vi "DataCollectTLSubs.vi"() -> ()   [LabVIEW 2009]
uses:
  BaudRateSelector.ctl
  <vilib>/Platform/TimedLoop/XDataNode/XDataNode.xnode
  <vilib>/Platform/TimedLoop/XDataNode/loadlvalarms.vi
  <vilib>/Platform/TimedLoop/XDataNode/timing_clust.ctl
  <vilib>/Platform/TimedLoop/XDataNode/nitl_modes.ctl
  <vilib>/Platform/TimedLoop/XDataNode/wakeup.ctl
  <vilib>/Platform/TimedLoop/scheduler/LVUserAPI/_suppVIs/Create_1kHz_TSource.vi
  <vilib>/Platform/TimedLoop/XDataNode/XDNodeRunTimeDep.lvlib
  <vilib>/Instr/_visa.llb/VISA Configure Serial Port (Instr).vi
panel:
  out "Sensor Names":string[](array[string])
  out "Degrees":dbl[](array[numeric]) format="%7.2f"
  in  "LH Calibration File":path
  out "Raw Data":u8[](array[numeric])
  out "Array 2":u32[](array[numeric])
  in  "Sampling Frequency (Hz)":u32 max=120 step=1
  in  "RH COM Port":refnum<visa-resource-name>="COM2"
  in  "LH COM Port":refnum<visa-resource-name>="COM1"
  out "Titles":string[](array[string])
  out "In queue":i32
  out "Interpreted Values":sgl[](array[numeric]) format="%.2f"
  out "Array":u32[](array[numeric])
  in  "stop":bool
  in  "Parity":enum16{"None", "Odd", "Even", "Mark", "Space"}(ring)
  in  "Data Bits":u16=8 min=7 max=8 step=1
  in  "Baud Rate":T1=115200 items=["1200"=1200, "2400"=2400, "4800"=4800, "9600"=9600, "19200"=19200, "38400"=38400, "57600"=57600, "115200"=115200]
  in  "COM Port":refnum<visa-resource-name>="COM3"
  # "Polhemus Serial Information"
  # "If Data Bits = 8, Parity must be \"None\""
  # "0 = As fast as possible"
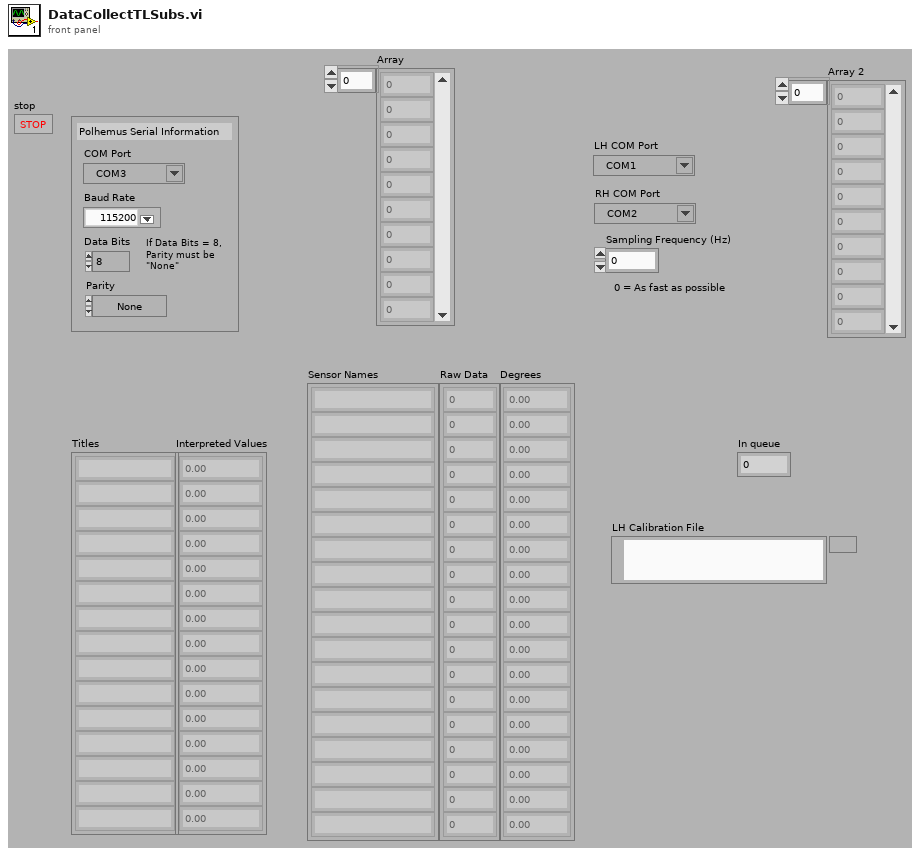
[diagram p1: front panel]
types:
  T1 = typedef "BaudRateSelector.ctl" = u32
  T2 = cluster{"#Bytes":i32[], "Titles":string[], "Format":enum16{"ASCII", "Binary"}, "Units":enum16{"Inches", "Centimeters"}, "Station State":bool[], "#Line Feeds":i32}
  T3 = typedef "XDNodeRunTimeDep.lvlib/timing_clust.ctl" = cluster{"Expected End [f-1]":u64, "Actual End [f-1]":u64, "Finished Late? [f-1]":bool, "Expected End [i-1]":u64, "Actual End [i-1]":u64, "Finished Late? [i-1]":bool, "Expected Start [i]":u64, "Actual Start [i]":u64, "Expected Start [f]":u64, "Actual Start [f]":u64, "Source Name":string, "Structure Name":string, "Period":i64, "Deadline":i64, "Offset":i64, "Start":i64, "Priority":i32, "Timeout":i32, "Mode":T4, "Wakeup Reason":T5, "Error":errorcluster, "Source Type":string, "Secondary Source Type":string, "Global End Time":u64, "Global Start Time":u64, "Frame Duration":u64, "Iteration Duration":u64, "Assigned CPU":i32, "I/O Scan Engine Mode":u32}
  T4 = typedef "XDNodeRunTimeDep.lvlib/nitl_modes.ctl" = enum32{"No Change", "Process missed periods, maintain original phase", "Discard missed periods, maintain original phase", "Process missed periods, ignore original phase", "Discard missed periods, ignore original phase"}
  T5 = typedef "XDNodeRunTimeDep.lvlib/wakeup.ctl" = enum32{"Normal", "Aborted", "Asynchronous wakeup", "Timing source error", "Timed loop error", "Timeout"}
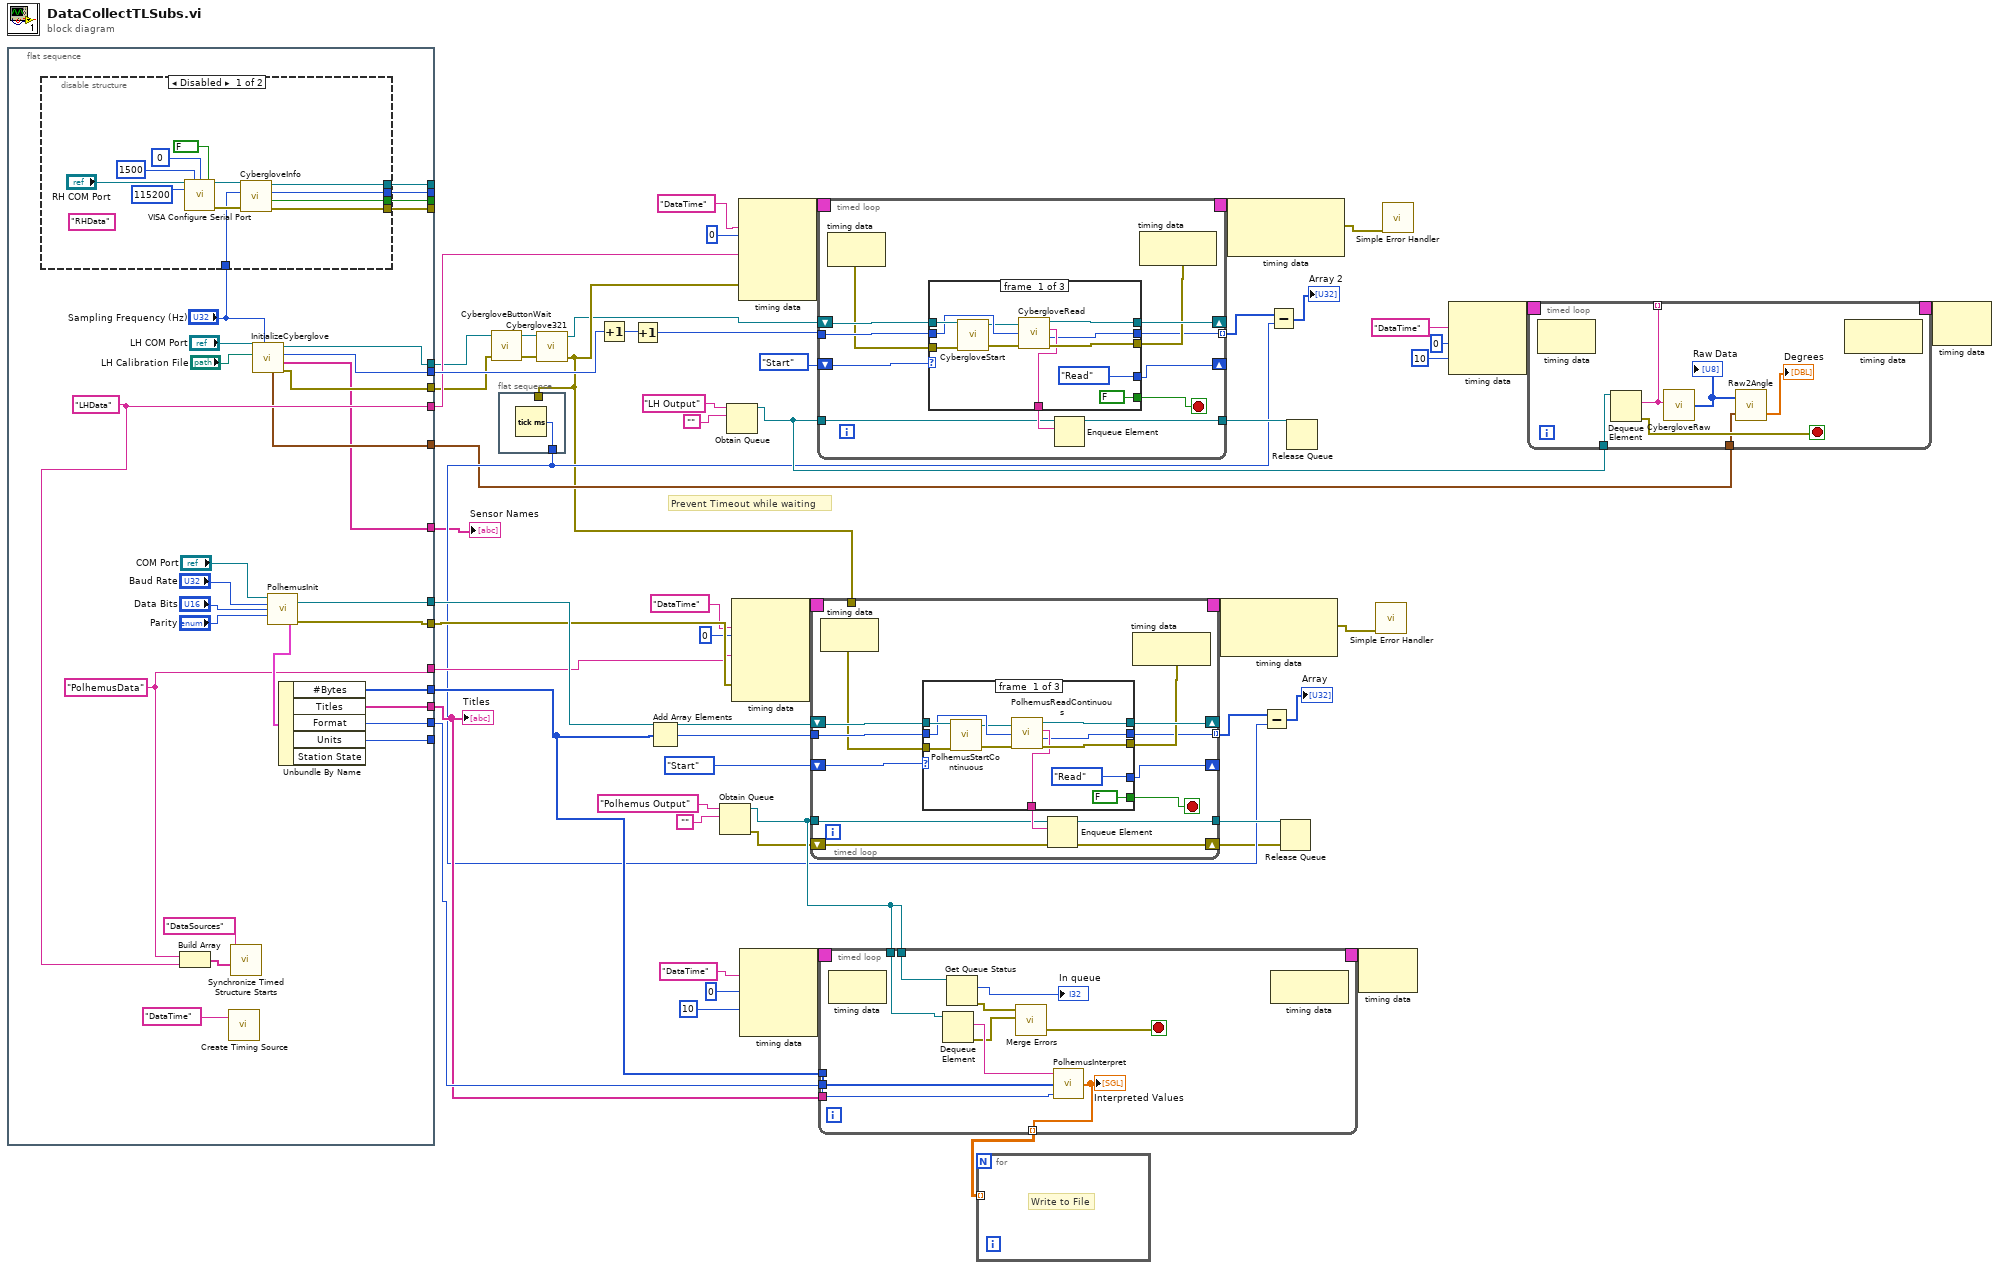
[diagram p0: block diagram]
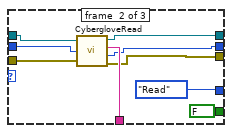
[diagram p2: hidden frame]
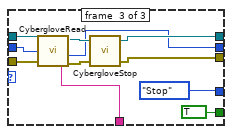
[diagram p3: hidden frame]
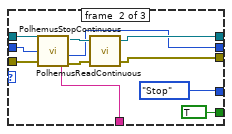
[diagram p5: hidden frame]
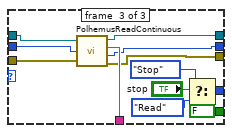
[diagram p6: hidden frame]
diagram:
  # "Prevent Timeout while waiting"
  n1 = flat-sequence {
    tunnel: [w80] -> w53
    tunnel: [w79] -> w52
    tunnel: [w78] -> w46
    tunnel: [w77] -> w41
    tunnel: [w76] -> _
    tunnel: [w75] -> w45
    tunnel: [w72] -> w39
    tunnel: [w69] -> w25
    tunnel: [w68] -> _
    tunnel: [w67] -> _
    tunnel: [w63] -> w24
    tunnel: [w66] -> w26
    tunnel: [w65] -> _
    tunnel: [w64] -> _
    tunnel: [w62] -> w23
    tunnel: [w60] -> w14
    tunnel: [w59] -> w1
    frame #0 {
      w69 = "LHData" ("Structure Name")
      w72 = "PolhemusData" ("Structure Name")
      n2 = disable-structure shown="Disabled" {
        disable-tunnel: [w90 _] -> w68
        disable-tunnel: [w89 _] -> w67
        disable-tunnel: [w88 _] -> w65
        disable-tunnel: [w87 _] -> w64
        disable-tunnel: "Sampling Frequency (Hz)" -> [w86 _]
        frame #0 {
          (unwired) "RHData" ("Structure Name")
          n3 = call-poly "VISA Configure Serial Port"("VISA resource name"="RH COM Port", "timeout (10sec)"=u32 1500, "termination char\n(0xA = '\\n' = LF)"=u8 0 ("termination char\n(0xA = '\\n' = LF)"), "Enable Termination\nChar (T)"=FALSE ("Enable Termination\nChar (T)"), "baud rate (9600)"=u32 115200) -> ("VISA resource name out"=w92:refnum<visa-resource-name>, "error out"=w91:errorcluster)  [unwired: 9 in]
          n4 = call "CybergloveInfo.vi"("error in (no error)"=w91, "Sampling Frequency (Hz)"=w86, "VISA resource name"=w92) -> ("error out"=w87:errorcluster, "RH?"=w89:bool, "#Sensors"=w90:i32, "VISA resource name out"=w88:refnum<visa-resource-name>)  [unwired: 3 in, 2 out]
        }
        frame #1 {
        }
      }
      n5 = Build Array(w72, w69) -> (w71:string[])
      n6 = call-poly <vilib>:"Create Timing Source.vi"("name (in)"="DataTime") -> ()  [unwired: 9 in, 2 out]
      n7 = call <vilib>:"Synchronize Timed Structure Starts.vi"("timed structure names"=w71, "synchronization group name"="DataSources") -> ()  [unwired: 8 in, 2 out]
      n8 = call "InitializeCyberglove.vi"("Sampling Frequency (0)"="Sampling Frequency (Hz)", "Calibration File"="LH Calibration File", "VISA resource name"="LH COM Port") -> ("error out"=w62:errorcluster, "Sensor Names"=w59:string[], "#Sensors"=w66:i32, "VISA resource name out"=w63:refnum<visa-resource-name>, "Calibration Array"=w60:cluster{"Offset":dbl, "Gain":dbl}[])  [unwired: 2 in]
      n9 = call "PolhemusInit.vi"("VISA resource name"="COM Port", "Baud Rate"="Baud Rate", "Data Bits"="Data Bits", "Parity"="Parity") -> ("VISA resource name out"=w80:refnum<visa-resource-name>, "Polhemus Info"=w81:T2, "error out"=w79:errorcluster)  [unwired: 9 in]
      n10 = Unbundle By Name(w81) -> ("#Bytes"=w78:i32[], "Titles"=w77:string[], "Format"=w75:enum16{"ASCII", "Binary"}, "Units"=w76:enum16{"Inches", "Centimeters"})  [unwired: 1 out]
    }
  }
  n11 = call "CybergloveButtonWait.vi"("error in (no error)"=w23, "VISA resource name"=w24) -> ("error out"=w21:errorcluster, "VISA resource name out"=w22:refnum<visa-resource-name>)  [unwired: 2 in]
  n12 = flat-sequence {
    tunnel: w13 -> [_]
    tunnel: [w98] -> w17
    frame #0 {
      n13 = Tick Count (ms)() -> (millisecond timer value=w98:u32)
    }
  }
  n14 = call "Cyberglove321.vi"("error in (no error)"=w21, "VISA resource name"=w22) -> ("error out"=w13:errorcluster, "VISA resource name out"=w12:refnum<visa-resource-name>)  [unwired: 2 in]
  n15 = Increment(x=w26) -> (x+1=w19:i32)
  n16 = Increment(x=w19) -> (x+1=w18:i32)
  n17 = Add Array Elements(numeric array=w46) -> (sum=w55:i32)
  n18 = Obtain Queue(name (unnamed)="Polhemus Output", element data type="") -> (queue out=w43:refnum<queue>, error out=w16:errorcluster)  [unwired: 3 in, 1 out]
  n19 = Obtain Queue(name (unnamed)="LH Output", element data type="") -> (queue out=w20:refnum<queue>)  [unwired: 3 in, 2 out]
  n20 = node-c288("DataTime" ("Source Name"), i64 0 ("Period"), w39, w52) -> (w57:T3)  [unwired: 1 in]
  n21 = node-c288("DataTime" ("Source Name"), i64 0 ("Period"), w25, w13) -> (w37:T3)  [unwired: 1 in]
  n22 = node-c288("DataTime" ("Source Name"), i64 0 ("Period"), 10 ("Priority")) -> (w11:T3)  [unwired: 1 in]
  n23 = timed-loop {
    timing: w57 -> [_]
    timing-out: [_] -> w56
    tunnel: w55 -> [w111]
    shift-right: [w107] -> _
    shift-left: enum16{"Start", "Read", "Stop"}."Start" -> [w110]
    shift-right: [w108] -> _
    shift-left: w53 -> [w112]
    tunnel: [w104] -> w50 mode=indexing
    tunnel: w43 -> [w102]
    tunnel: [w101] -> w44
    tunnel: w13 -> [_]
    shift-right: [w99] -> w15
    shift-left: w16 -> [w100]
    stop <- w106 stop-if-true
    n24 = node-c288() -> (w109:errorcluster)  [unwired: 1 in]
    n25 = case shown="\"Read\"" w110 {
      tunnel: w112 -> [w123 w130 w146]
      tunnel: [w116 w133 w145] -> w103
      tunnel: w111 -> [w121 w134 w144]
      tunnel: w109 -> [w122 w129 w137]
      tunnel: [w118 w126 w138] -> w108
      tunnel: [w117 w125 w136] -> w105
      tunnel: [enum16{"Start", "Read", "Stop"}."Read" enum16{"Start", "Read", "Stop"}."Stop" w140] -> w107
      tunnel: [FALSE TRUE FALSE] -> w106
      tunnel: [w113 w124 w135] -> w104
      frame #0 {
        n26 = call "PolhemusStartContinuous.vi"("error in (no error)"=w122, "VISA resource name"=w123) -> ("error out"=w119:errorcluster, "VISA resource name out"=w120:refnum<visa-resource-name>)  [unwired: 2 in]
        n27 = call "PolhemusReadContinuous.vi"("VISA resource name"=w120, "Byte Sum"=w121, "error in (no error)"=w119) -> ("VISA resource name out"=w118:refnum<visa-resource-name>, "Polhemus Output"=w116:string, "Time"=w113:u32, "error out"=w117:errorcluster)
      }
      frame #1 {
        n28 = call "PolhemusReadContinuous.vi"("VISA resource name"=w130, "Byte Sum"=w134, "error in (no error)"=w129) -> ("VISA resource name out"=w128:refnum<visa-resource-name>, "Polhemus Output"=w133:string, "Time"=w124:u32, "error out"=w127:errorcluster)
        n29 = call "PolhemusStopContinuous.vi"("error in (no error)"=w127, "VISA resource name"=w128) -> ("error out"=w125:errorcluster, "VISA resource name out"=w126:refnum<visa-resource-name>)  [unwired: 2 in]
      }
      frame #2 {
        n30 = call "PolhemusReadContinuous.vi"("VISA resource name"=w146, "Byte Sum"=w144, "error in (no error)"=w137) -> ("VISA resource name out"=w138:refnum<visa-resource-name>, "Polhemus Output"=w145:string, "Time"=w135:u32, "error out"=w136:errorcluster)
        n31 = Select(t=enum16{"Start", "Read", "Stop"}."Stop", s="stop", f=enum16{"Start", "Read", "Stop"}."Read") -> (s? t:f=w140:enum16{"Start", "Read", "Stop"})
      }
    }
    n32 = Enqueue Element(queue=w102, element=w103, error in (no error)=w100) -> (queue out=w101:refnum<queue>, error out=w99:errorcluster)  [unwired: 1 in, 1 out]
    n33 = node-c288(w105) -> ()  [unwired: 1 out]
  }
  n34 = timed-loop {
    timing: w37 -> [_]
    timing-out: [_] -> w36
    tunnel: w18 -> [w162]
    shift-right: [w158] -> _
    shift-left: enum16{"Start", "Read", "Stop"}."Start" -> [w161]
    shift-right: [w159] -> _
    shift-left: w12 -> [w163]
    tunnel: [w155] -> w33 mode=indexing
    tunnel: w20 -> [w153]
    tunnel: [w152] -> w29
    stop <- w157 stop-if-true
    n35 = node-c288() -> (w160:errorcluster)  [unwired: 1 in]
    n36 = case shown="\"Read\"" w161 {
      tunnel: w163 -> [w174 w183 w190]
      tunnel: [w167 w182 w193] -> w154
      tunnel: w162 -> [w172 w181 w194]
      tunnel: w160 -> [w173 w178 w189]
      tunnel: [w169 w179 w186] -> w159
      tunnel: [w168 w177 w185] -> w156
      tunnel: [enum16{"Start", "Read", "Stop"}."Read" enum16{"Start", "Read", "Stop"}."Read" enum16{"Start", "Read", "Stop"}."Stop"] -> w158
      tunnel: [FALSE FALSE TRUE] -> w157
      tunnel: [w164 w176 w184] -> w155
      frame #0 {
        n37 = call "CybergloveStart.vi"("error in (no error)"=w173, "VISA resource name"=w174) -> ("error out"=w170:errorcluster, "VISA resource name out"=w171:refnum<visa-resource-name>)  [unwired: 2 in]
        n38 = call "CybergloveRead.vi"("VISA resource name"=w171, "Bytes"=w172, "error in (no error)"=w170) -> ("VISA resource name out"=w169:refnum<visa-resource-name>, "Cyberglove Output"=w167:string, "Time"=w164:u32, "error out"=w168:errorcluster)
      }
      frame #1 {
        n39 = call "CybergloveRead.vi"("VISA resource name"=w183, "Bytes"=w181, "error in (no error)"=w178) -> ("VISA resource name out"=w179:refnum<visa-resource-name>, "Cyberglove Output"=w182:string, "Time"=w176:u32, "error out"=w177:errorcluster)
      }
      frame #2 {
        n40 = call "CybergloveRead.vi"("VISA resource name"=w190, "Bytes"=w194, "error in (no error)"=w189) -> ("VISA resource name out"=w188:refnum<visa-resource-name>, "Cyberglove Output"=w193:string, "Time"=w184:u32, "error out"=w187:errorcluster)
        n41 = call "CybergloveStop.vi"("error in (no error)"=w187, "VISA resource name"=w188) -> ("error out"=w185:errorcluster, "VISA resource name out"=w186:refnum<visa-resource-name>)  [unwired: 2 in]
      }
    }
    n42 = Enqueue Element(queue=w153, element=w154) -> (queue out=w152:refnum<queue>)  [unwired: 2 in, 2 out]
    n43 = node-c288(w156) -> ()  [unwired: 1 out]
  }
  n44 = timed-loop {
    tunnel: w43 -> [w209]
    tunnel: w46 -> [w207]
    tunnel: w45 -> [w206]
    tunnel: w43 -> [w205]
    tunnel: [w200] -> w42 mode=indexing
    tunnel: w41 -> [_]
    timing: w11 -> [_]
    timing-out: [_] -> w10
    stop <- w203 stop-if-true
    n45 = node-c288() -> ()  [unwired: 1 in, 1 out]
    n46 = Dequeue Element(queue=w209) -> (element=w208:string, error out=w202:errorcluster)  [unwired: 2 in, 2 out]
    n47 = Get Queue Status(queue=w205) -> (# pending remove=→"In queue":i32, error out=w201:errorcluster)  [unwired: 2 in, 6 out]
    n48 = call <vilib>:"Merge Errors.vi"("error in 2 (no error)"=w202, "error in 1 (no error)"=w201) -> ("error out"=w203:errorcluster)  [unwired: 5 in]
    n49 = call "PolhemusInterpret.vi"("Format"=w206, "#Bytes"=w207, "Polhemus Output"=w208) -> ("Interpreted Values"=w200:sgl[])  [unwired: 1 in]
    "Interpreted Values" <- w200
    n50 = node-c288() -> ()  [unwired: 1 in, 1 out]
  }
  n51 = for {
    tunnel: w42 -> [_] mode=indexing
    # "Write to File"
  }
  n52 = node-c288(w56) -> (w54:errorcluster)  [unwired: 1 out]
  n53 = node-c288(w36) -> (w35:errorcluster)  [unwired: 1 out]
  n54 = Subtract(x=w50, y=w17) -> (x-y=→"Array":u32[])
  n55 = Subtract(x=w33, y=w17) -> (x-y=→"Array 2":u32[])
  n56 = Release Queue(queue=w44, error in (no error)=w15) -> ()  [unwired: 1 in, 3 out]
  n57 = Release Queue(queue=w29) -> ()  [unwired: 2 in, 3 out]
  n58 = node-c288(w10) -> ()  [unwired: 1 out]
  n59 = call <vilib>:"Simple Error Handler.vi"("error in (no error)"=w54) -> ()  [unwired: 4 in, 5 out]
  n60 = call <vilib>:"Simple Error Handler.vi"("error in (no error)"=w35) -> ()  [unwired: 4 in, 5 out]
  n61 = node-c288("DataTime" ("Source Name"), i64 0 ("Period"), 10 ("Priority")) -> (w6:T3)
  n62 = timed-loop {
    tunnel: w20 -> [w217]
    tunnel: [w215] -> _ mode=indexing
    tunnel: w14 -> [w214]
    timing: w6 -> [_]
    timing-out: [_] -> w5
    stop <- w216 stop-if-true
    n63 = node-c288() -> ()  [unwired: 1 in, 1 out]
    n64 = Dequeue Element(queue=w217) -> (element=w215:string, error out=w216:errorcluster)  [unwired: 2 in, 2 out]
    n65 = call "CybergloveRaw.vi"("Cyberglove Out"=w215) -> ("Raw Data"=w213:u8[])
    "Raw Data" <- w213
    n66 = call "Raw2Angle.vi"("Calibration"=w214, "Raw Data"=w213) -> ("Degrees"=→"Degrees":dbl[])  [unwired: 1 out]
    n67 = node-c288() -> ()  [unwired: 1 in, 1 out]
  }
  n68 = node-c288(w5) -> ()  [unwired: 1 out]
  "Titles" <- w41
  "Sensor Names" <- w1
